vi "Main On Compile Action VI.vi"(8 "error in (no error)":errorcluster, 11 "Device Item Ref in":T1 format="%.0x") -> (0 "error out":errorcluster)   [LabVIEW 2013, in "PWM System Explorer.lvlib"]
uses:
  PWM System Explorer.lvlib
  <vilib>/NI Veristand/Custom Device API/Custom Device Item Ref.ctl
  Shared/Types/PWM data.ctl
  Shared/Types/PWM out info.ctl
  Shared/Types/PWM in info.ctl
  NationalInstruments.VeriStand.SystemStorage
  Shared/Constants.vi
  <vilib>/NI Veristand/Custom Device API/Get Item Property (Variant).vi
  <vilib>/NI Veristand/Custom Device API/Set Item Property (Variant).vi
  <vilib>/NI Veristand/Custom Device API/Custom Device API.lvlib
  Shared/PWM Shared.lvlib
  <vilib>/NI Veristand/Custom Device Tools/Custom Device Utility Library/Custom Device Utility Library.lvlib
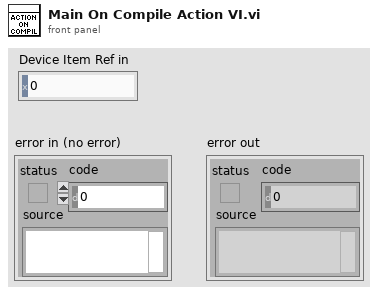
[diagram p1: front panel]
types:
  T1 = typedef "Custom Device API.lvlib/Custom Device Item Ref.ctl" = u64
  T2 = typedef "PWM Shared.lvlib/PWM data.ctl" = cluster{"PWM out(added)":T3[], "PWM out(not added)":T3[], "PWM in(added)":T4[]}
  T3 = typedef "PWM Shared.lvlib/PWM out info.ctl" = cluster{"PWM out name":string, "buffer index (Duty cycle)":i32, "buffer index (Frequency)":i32, "Init Frequency":dbl, "Init Duty Cycle":dbl}
  T4 = typedef "PWM Shared.lvlib/PWM in info.ctl" = cluster{"PWM in name":string, "buffer index (Duty cycle)":i32, "buffer index (Frequency)":i32, "Timeout name":string, "Timeout val":dbl}
  T5 = typedef "Custom Device API.lvlib/Custom Device Pointer.ctl" = refnum<k24>
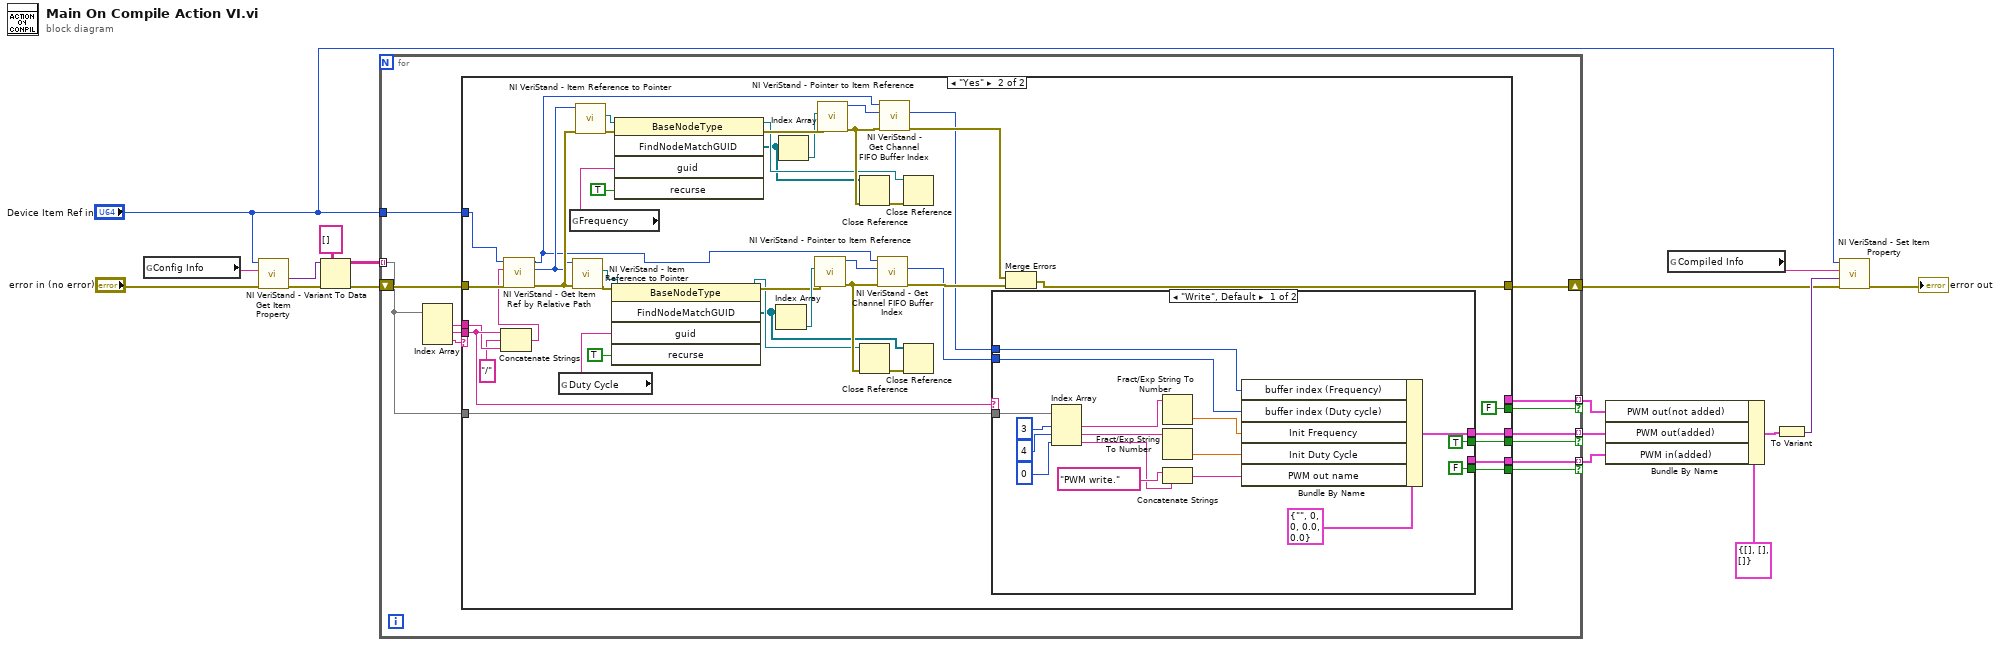
[diagram p0: block diagram]
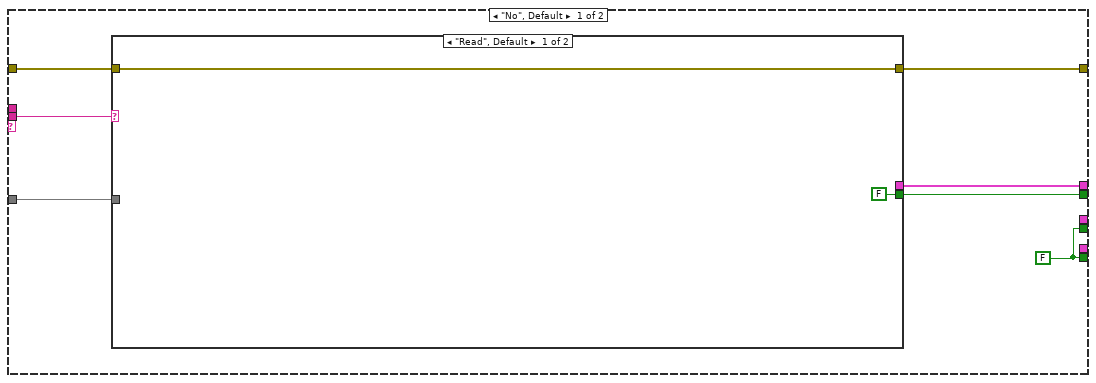
[diagram p2: hidden frame]
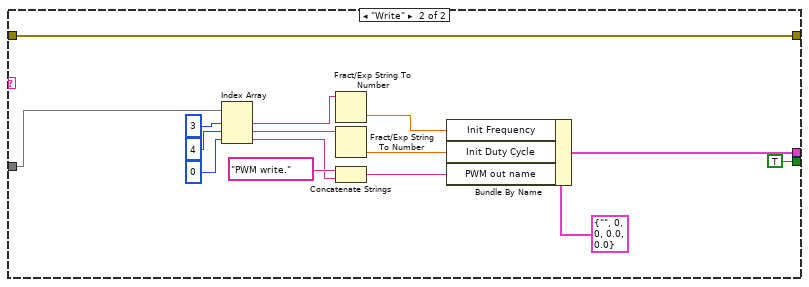
[diagram p3: hidden frame]
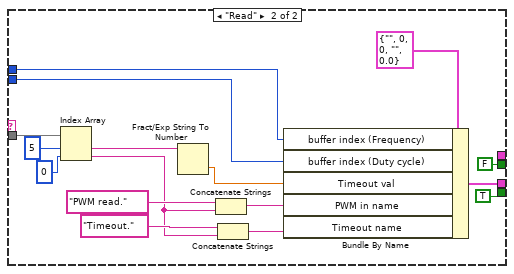
[diagram p4: hidden frame]
diagram:
  n1 = global read "Constants.vi" "Config Info"() -> (w17:string)
  n2 = call-poly <vilib>:"NI VeriStand - Get Item Property.vi"("error in (no error)"="error in (no error)", "Property Name"=w17, "Item Ref in"="Device Item Ref in") -> ("error out"=w14:errorcluster, "Value"=w16:variant)  [unwired: 5 in, 2 out]
  n3 = Variant To Data(error in=w14, type=string[][] [] ("Control Info"), Variant=w16) -> (data=w12:string[][], error out=w11:errorcluster)
  n4 = for {
    tunnel: w12 -> [w18] mode=indexing
    shift-right: [w29] -> w4
    shift-left: w11 -> [w30]
    tunnel: "Device Item Ref in" -> [w28]
    tunnel: [w25] -> w8 mode=indexing if=w24
    tunnel: [w23] -> w9 mode=indexing if=w22
    tunnel: [w21] -> w10 mode=indexing if=w20
    n5 = Index Array(array=w18) -> (element #1=w19:string, element #2=w26:string, element #3=w27:string)  [unwired: 3 in]
    n6 = case shown="\"Yes\"" w27 {
      tunnel: w30 -> [w36 w60]
      tunnel: w18 -> [w37 w66]
      tunnel: [w35 w67] -> w29
      tunnel: w28 -> [_ w58]
      tunnel: w26 -> [w34 w63]
      tunnel: [_ w72] -> w25
      tunnel: [w31 w71] -> w24
      tunnel: [_ w70] -> w23
      tunnel: [w31 w69] -> w22
      tunnel: [w33 _] -> w21
      tunnel: [w32 FALSE] -> w20
      tunnel: w19 -> [_ w62]
      frame "No", Default {
        w31 = FALSE
        n7 = case shown="\"Read\", Default" w34 {
          tunnel: w37 -> [_ w49]
          tunnel: [w39 w54] -> w35
          tunnel: w36 -> [w39 w54]
          tunnel: [_ w46] -> w33
          tunnel: [FALSE TRUE] -> w32
          frame "Read", Default {
          }
          frame "Write" {
            n8 = Index Array(array=w49, index #1=3 ("index"), index #2=4 ("index"), index #3=0 ("index")) -> (element #1=w51:string, element #2=w50:string, element #3=w40:string)
            n9 = Fract/Exp String To Number(string=w51) -> (number=w47:dbl)  [unwired: 3 in, 1 out]
            n10 = Fract/Exp String To Number(string=w50) -> (number=w48:dbl)  [unwired: 3 in, 1 out]
            n11 = Concatenate Strings("PWM write." ("PWM out name"), w40) -> (w43:string)
            n12 = Bundle By Name(cluster=T3 {"PWM out name"="", "buffer index (Duty cycle)"=0, "buffer index (Frequency)"=0, "Init Frequency"=0.0, "Init Duty Cycle"=0.0} ("PWM out info"), "Init Frequency"=w47, "Init Duty Cycle"=w48, "PWM out name"=w43) -> (w46:T3)
          }
        }
      }
      frame "Yes" {
        n13 = Concatenate Strings(w63, "/" ("string"), w62) -> (w57:string)
        n14 = call <vilib>:"NI VeriStand - Get Item Ref by Relative Path.vi"("error in"=w60, "Relative Item Path"=w57, "Section Ref in"=w58) -> ("error out"=w59:errorcluster, "Item Ref"=w56:T1, "Section Ref out"=w55:T1)  [unwired: 5 in, 1 out]
        n15 = global read "Constants.vi" "Duty Cycle"() -> (w83:string)
        n16 = global read "Constants.vi" "Frequency"() -> (w84:string)
        n17 = call <vilib>:"NI VeriStand - Item Reference to Pointer.vi"("error in (no error)"=w59, "Item Ref in"=w56) -> ("error out"=w94:errorcluster, "Node Pointer"=w95:T5)  [unwired: 6 in, 2 out]
        n18 = call <vilib>:"NI VeriStand - Item Reference to Pointer.vi"("error in (no error)"=w59, "Item Ref in"=w56) -> ("error out"=w87:errorcluster, "Node Pointer"=w86:T5)  [unwired: 6 in, 2 out]
        n19 = invoke class="BaseNodeType" method="FindNodeMatchGUID"(reference=w95, error in=w94, "guid"=w83, "recurse"=TRUE) -> (reference out=w76:T5, error out=w92:errorcluster, "FindNodeMatchGUID"=w75:refnum<k24>[])  [unwired: 1 in, 2 out]
        n20 = invoke class="BaseNodeType" method="FindNodeMatchGUID"(reference=w86, error in=w87, "guid"=w84, "recurse"=TRUE) -> (reference out=w74:T5, error out=w89:errorcluster, "FindNodeMatchGUID"=w73:refnum<k24>[])  [unwired: 1 in, 2 out]
        n21 = Index Array(array=w75) -> (element=w93:refnum<k24>)  [unwired: 1 in]
        n22 = Index Array(array=w73) -> (element=w88:refnum<k24>)  [unwired: 1 in]
        n23 = call <vilib>:"NI VeriStand - Pointer to Item Reference.vi"("error in (no error)"=w92, "Node Pointer"=w93) -> ("error out"=w80:errorcluster, "Item Ref out"=w79:T1)  [unwired: 8 in]
        n24 = call <vilib>:"NI VeriStand - Pointer to Item Reference.vi"("error in (no error)"=w89, "Node Pointer"=w88) -> ("error out"=w81:errorcluster, "Item Ref out"=w82:T1)  [unwired: 8 in]
        n25 = Close Reference(reference=w73, error in (no error)=w81) -> (error out=w90:errorcluster)
        n26 = Close Reference(reference=w76, error in (no error)=w80) -> (error out=w91:errorcluster)
        n27 = call <vilib>:"NI VeriStand - Get Channel FIFO Buffer Index.vi"("error in"=w80, "Channel Ref"=w79, "Device Ref in"=w55) -> ("error out"=w78:errorcluster, "Channel FIFO Buffer Index"=w64:i32)  [unwired: 4 in, 3 out]
        n28 = call <vilib>:"NI VeriStand - Get Channel FIFO Buffer Index.vi"("error in"=w81, "Channel Ref"=w82, "Device Ref in"=w55) -> ("error out"=w77:errorcluster, "Channel FIFO Buffer Index"=w65:i32)  [unwired: 4 in, 3 out]
        n29 = Close Reference(reference=w74, error in (no error)=w90) -> ()  [unwired: 1 out]
        n30 = Close Reference(reference=w75, error in (no error)=w91) -> ()  [unwired: 1 out]
        n31 = case shown="\"Write\", Default" w63 {
          tunnel: w66 -> [w113 w129]
          tunnel: w64 -> [w103 w120]
          tunnel: w65 -> [w104 w121]
          tunnel: [_ w114] -> w72
          tunnel: [FALSE TRUE] -> w71
          tunnel: [w97 _] -> w70
          tunnel: [TRUE FALSE] -> w69
          frame "Write", Default {
            n32 = Index Array(array=w113, index #1=3 ("index"), index #2=4 ("index"), index #3=0 ("index")) -> (element #1=w109:string, element #2=w108:string, element #3=w98:string)
            n33 = Fract/Exp String To Number(string=w109) -> (number=w105:dbl)  [unwired: 3 in, 1 out]
            n34 = Fract/Exp String To Number(string=w108) -> (number=w106:dbl)  [unwired: 3 in, 1 out]
            n35 = Concatenate Strings("PWM write." ("PWM out name"), w98) -> (w107:string)
            n36 = Bundle By Name(cluster=T3 {"PWM out name"="", "buffer index (Duty cycle)"=0, "buffer index (Frequency)"=0, "Init Frequency"=0.0, "Init Duty Cycle"=0.0} ("PWM out info"), "buffer index (Frequency)"=w104, "buffer index (Duty cycle)"=w103, "Init Frequency"=w105, "Init Duty Cycle"=w106, "PWM out name"=w107) -> (w97:T3)
          }
          frame "Read" {
            n37 = Index Array(array=w129, index #1=5 ("index"), index #2=0 ("index")) -> (element #1=w123:string, element #2=w116:string)
            n38 = Fract/Exp String To Number(string=w123) -> (number=w122:dbl)  [unwired: 3 in, 1 out]
            n39 = Concatenate Strings("PWM read." ("PWM out name"), w116) -> (w115:string)
            n40 = Concatenate Strings("Timeout." ("PWM out name"), w116) -> (w125:string)
            n41 = Bundle By Name(cluster=T4 {"PWM in name"="", "buffer index (Duty cycle)"=0, "buffer index (Frequency)"=0, "Timeout name"="", "Timeout val"=0.0} ("PWM in info"), "buffer index (Frequency)"=w121, "buffer index (Duty cycle)"=w120, "Timeout val"=w122, "PWM in name"=w115, "Timeout name"=w125) -> (w114:T4)
          }
        }
        n42 = Merge Errors(w77, w78) -> (w67:errorcluster)
      }
    }
  }
  n43 = Bundle By Name(cluster=T2 {"PWM out(added)"=[], "PWM out(not added)"=[], "PWM in(added)"=[]} ("PWM out(added)"), "PWM out(not added)"=w10, "PWM out(added)"=w9, "PWM in(added)"=w8) -> (w7:T2)
  n44 = global read "Constants.vi" "Compiled Info"() -> (w5:string)
  n45 = To Variant(anything=w7) -> (Variant=w6:variant)
  n46 = call-poly <vilib>:"NI VeriStand - Set Item Property.vi"("error in (no error)"=w4, "Value"=w6, "Property Name"=w5, "Item Ref in"="Device Item Ref in") -> ("error out"=→"error out":errorcluster)  [unwired: 5 in, 2 out]
